vi "set_1550_nm.vi"(9 "error in (no error)":errorcluster, 10 "Visa Session":refnum<visa-resource-name>="USB0::0x0BD3::0x0333::NI-VISA-30004::RAW", 11 "wave nm":string="1550") -> (1 "Device Response":string="*\n", 2 "dup Visa Session":refnum<visa-resource-name>="USB0::0x0BD3::0x0333::NI-VISA-30004::RAW", 8 "error out":errorcluster)   [LabVIEW 2018]
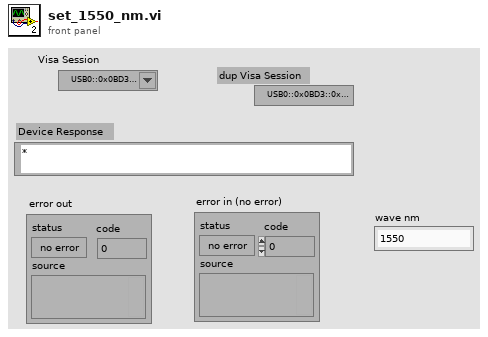
[diagram p1: front panel]
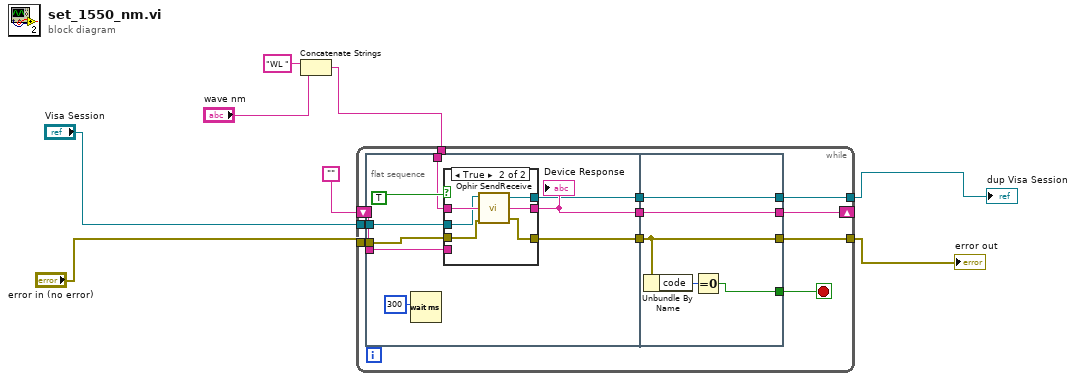
[diagram p0: block diagram]
diagram:
  n1 = Concatenate Strings("WL " ("string"), "wave nm") -> (w3:string)
  n2 = while {
    tunnel: [w16] -> w5
    tunnel: [w14] -> w7
    shift-left: "" -> [w18]
    shift-right: [w19] -> _
    tunnel: "error in (no error)" -> [w15]
    tunnel: "Visa Session" -> [w17]
    tunnel: w3 -> [w13]
    stop <- w9 stop-if-true
    n3 = flat-sequence {
      tunnel: w18 -> [w26]
      tunnel: w17 -> [w25]
      tunnel: w15 -> [w22]
      tunnel: w13 -> [w20]
      tunnel: [w27] -> w12
      tunnel: [w24] -> w11
      tunnel: [w21] -> w10
      tunnel: [w39] -> w14
      tunnel: [w41] -> w16
      tunnel: [w42] -> w19
      tunnel: w12 -> [w42]
      tunnel: w11 -> [w41]
      tunnel: w10 -> [w39]
      tunnel: [w38] -> w9
      frame #0 {
        n4 = Wait (ms)(milliseconds to wait=u32 300) -> ()  [unwired: 1 out]
        n5 = case shown="True" TRUE ("Send Command (Enter)") {
          tunnel: w20 -> [_ w37]
          tunnel: [w31 w36] -> w27
          tunnel: w26 -> [w31 _]
          tunnel: w25 -> [w30 w35]
          tunnel: w22 -> [w29 w34]
          tunnel: [w29 w33] -> w21
          tunnel: [w30 w32] -> w24
          frame False {
          }
          frame True {
            n6 = call "Ophir SendReceive.vi"("error in (no error)"=w34, "Command"=w37, "Visa Session"=w35) -> ("error out"=w33:errorcluster, "Frame Output"=w36:string, "dup Visa Session"=w32:refnum<visa-resource-name>)
          }
        }
        "Device Response" <- w27
      }
      frame #1 {
        n7 = Unbundle By Name(w39) -> ("code"=w40:i32)
        n8 = Equal To 0?(x=w40) -> (x = 0?=w38:bool)
      }
    }
  }
  "error out" <- w7
  "dup Visa Session" <- w5
